vi "oa_Regulate Even Angle Signal (N Channels).vi"(5 "# of ch":i32, 7 "reset?":bool, 8 "samples/rev":dbl, 9 "offset":dbl, 10 "time stamps":dbl[](array[numeric]) format="%.2f", 11 "Data":dbl[][](array[numeric]) format="%.2f") -> (0 "actual max order":dbl, 2 "even-angle position info":T1, 3 "even-angle signals":cluster{"r0":dbl, "dr":dbl, "Y":dbl[]}[](array[cluster]) {"r0" format="%.2p"; "dr" format="%.2p"; "Y" format="%.2f"})   [LabVIEW 2017, in "SoundVib_Resampling.lvlib"]
uses:
  <vilib>/addons/Sound and Vibration/Order Analysis/Resample Order Tracking/SoundVib_Resampling.lvlib
  <vilib>/addons/Sound and Vibration/Order Analysis/Misc/OAT Position Info.ctl
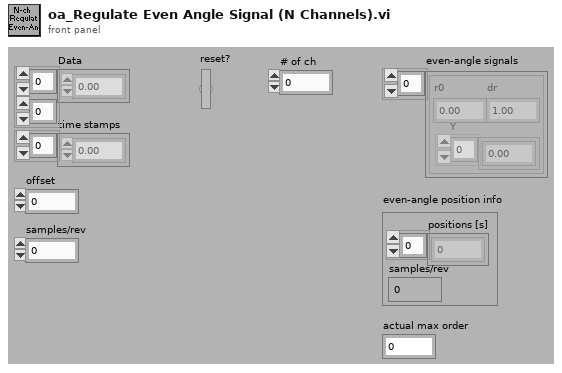
[diagram p1: front panel]
types:
  T1 = typedef "OAT Position Info.ctl" = cluster{"positions [s]":dbl[], "samples/rev":dbl}
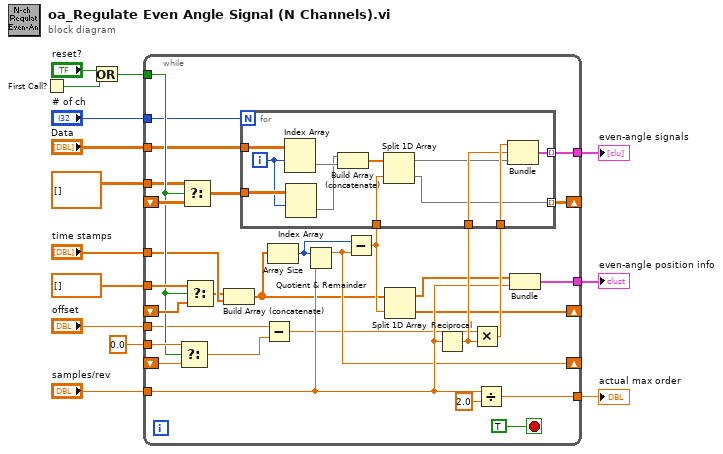
[diagram p0: block diagram]
diagram:
  n1 = First Call?() -> (First Call?: T/F=w7:bool)
  n2 = Or(x="reset?", y=w7) -> (x .or. y?=w8:bool)
  n3 = while {
    tunnel: "time stamps" -> [w32]
    tunnel: "offset" -> [w24]
    tunnel: "samples/rev" -> [w40]
    tunnel: "Data" -> [w17]
    shift-right: [w29] -> _
    shift-left: _ -> [w39]
    tunnel: dbl[] [] ("time stamps") -> [w37]
    tunnel: w8 -> [w34]
    shift-right: [w28] -> _
    shift-left: _ -> [w38]
    shift-right: [w26] -> _
    shift-left: _ -> [w36]
    tunnel: 0.0 ("t") -> [w35]
    tunnel: [w22] -> w1
    tunnel: [w21] -> w4
    tunnel: [w20] -> w5
    tunnel: dbl[][] [] ("time stamps") -> [w18]
    tunnel: "# of ch" -> [w15]
    stop <- TRUE stop-if-true
    n4 = Select(t=w35, s=w34, f=w36) -> (s? t:f=w23:dbl)
    n5 = Select(t=w18, s=w34, f=w38) -> (s? t:f=w16:dbl[][])
    n6 = Select(t=w37, s=w34, f=w39) -> (s? t:f=w31:dbl[])
    n7 = Build Array (concatenate)(w31, w32) -> (w19:dbl[])
    n8 = Subtract(x=w24, y=w23) -> (x-y=w25:dbl)
    n9 = Array Size(array=w19) -> (size(s)=w33:i32)
    n10 = Quotient & Remainder(x=w33, y=w40) -> (x-y*floor(x/y)=w26:dbl)  [unwired: 1 out]
    n11 = Subtract(x=w33, y=w26) -> (x-y=w30:dbl)
    n12 = Split 1D Array(array=w19, index=w30) -> (first subarray=w27:dbl[], second subarray=w29:dbl[])
    n13 = Reciprocal(x=w40) -> (1/x=w43:dbl)
    n14 = Multiply(x=w25, y=w43) -> (x*y=w44:dbl)
    n15 = for {
      N: w15 -> [_]
      tunnel: w44 -> [w56]
      tunnel: w43 -> [w55]
      tunnel: w30 -> [w54]
      tunnel: [w53] -> w28 mode=indexing
      tunnel: [w51] -> w22 mode=indexing
      tunnel: w17 -> [w50]
      tunnel: w16 -> [w46]
      i -> [w45]
      n16 = Index Array(array=w50, index (row)=w45) -> (element=w48:dbl[])  [unwired: 1 in]
      n17 = Index Array(array=w46, index (row)=w45) -> (element=w47:dbl[])  [unwired: 1 in]
      n18 = Build Array (concatenate)(w47, w48) -> (w49:dbl[])
      n19 = Split 1D Array(array=w49, index=w54) -> (first subarray=w52:dbl[], second subarray=w53:dbl[])
      n20 = Bundle(w56, w55, w52) -> (w51:cluster{dbl, dbl, dbl[]})  [unwired: 1 in]
    }
    n21 = Divide(x=w40, y=2.0) -> (x/y=w20:dbl)
    n22 = Bundle(w27, "samples/rev"=w40) -> (w21:cluster{dbl[], "samples/rev":dbl})  [unwired: 1 in]
  }
  "even-angle position info" <- w4
  "actual max order" <- w5
  "even-angle signals" <- w1
